vi "VI 1.vi"() -> ()   [LabVIEW 2020]
uses:
  <vilib>/express/express analysis/Spectral/Block/exnSpectralBlock spectral measurements RMS poly.vi
  <vilib>/express/express analysis/Spectral/Block/exnSpectralBlock spectral measurements RMS DDT.vi
  <vilib>/express/express analysis/Spectral/XNode/ExpressSpectralMeasurementsBlockNode.xnode
panel:
  out "Minimum":dbl
  out "Maksimum":dbl
  out "RMS":dbl
  out "Specific Harmonic Level":dbl
  out "THD":dbl
  out "SINAD":dbl
  out "Przebieg FFT":dynamicdata(graph)
  in  "Numer Harmonicznej":dbl=2.0 min=2.0 step=1.0
  in  "Faza 4":dbl min=0.0 step=0.1
  in  "Amplituda 4":dbl step=0.1
  in  "Numer Harmonicznej":dbl=2.0 min=2.0 step=1.0
  in  "Faza 3":dbl min=0.0 step=0.1
  in  "Amplituda 3":dbl step=0.1
  in  "Numer Harmonicznej":dbl=2.0 min=2.0 step=1.0
  in  "Faza 2":dbl min=0.0 step=0.1
  in  "Amplituda 2":dbl=0.1 step=0.1
  in  "Faza 1":dbl=0.1 min=0.0 step=0.1
  in  "Amplituda 1":dbl=0.1 step=0.1
  in  "Czestotliwosc Bazowa":dbl=1.0 min=1.0 step=0.1
  out "Przebieg Sygnalu":dynamicdata(graph)
  in  "Stop":bool
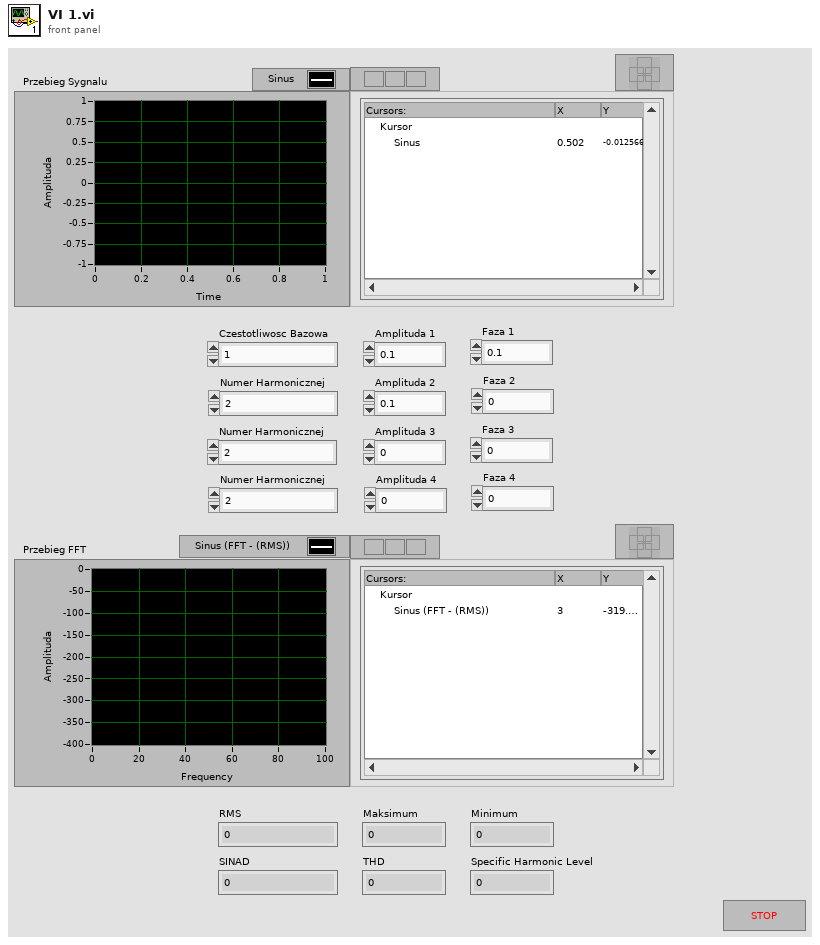
[diagram p1: front panel]
types:
  T1 = cluster{"averaging mode":u16, "weighting mode":u16, "number of averages":u32}
  T2 = cluster{"dB On (F)":bool, "unwrap phase (F)":bool, "convert to degree (F)":bool}
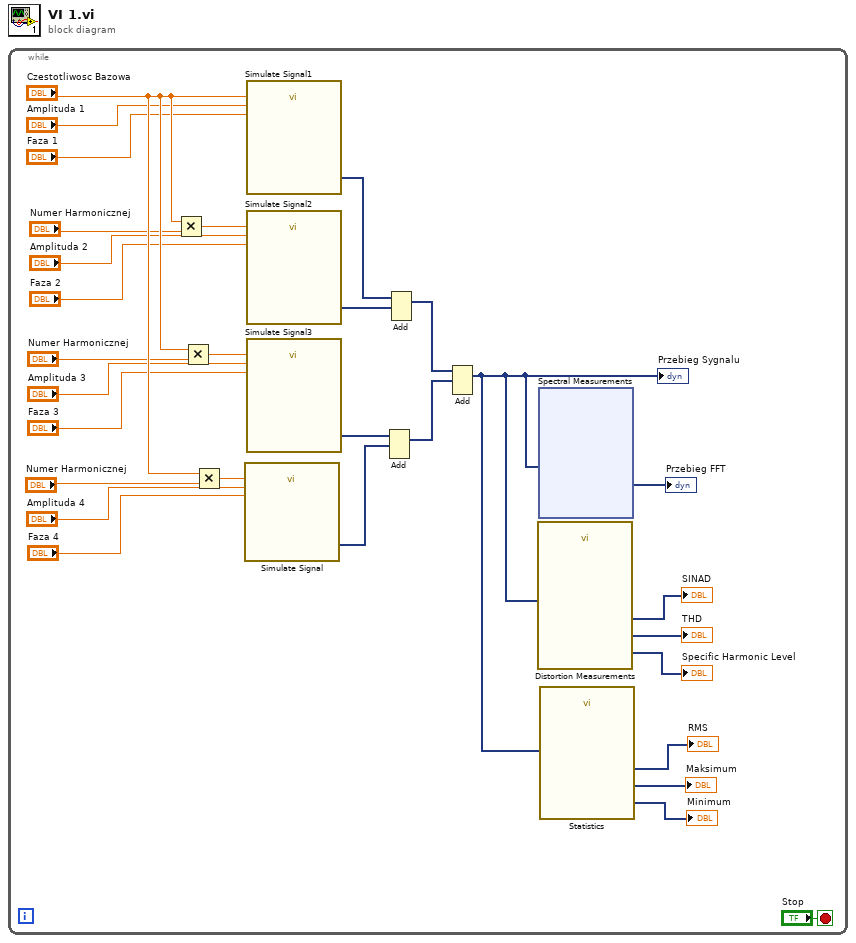
[diagram p0: block diagram]
diagram:
  n1 = while {
    stop <- "Stop" stop-if-true
    n2 = Multiply(x="Czestotliwosc Bazowa", y="Numer Harmonicznej") -> (x*y=w26:dbl)
    n3 = Multiply(x="Czestotliwosc Bazowa", y="Numer Harmonicznej") -> (x*y=w25:dbl)
    n4 = Multiply(x="Czestotliwosc Bazowa", y="Numer Harmonicznej") -> (x*y=w21:dbl)
    n5 = call "Simulate Signal"("Frequency"=w21, "Amplitude"="Amplituda 4", "Phase"="Faza 4") -> ("Harmoniczna3"=w23:dynamicdata)  [unwired: 11 in, 1 out]
    n6 = call "Simulate Signal1"("Frequency"="Czestotliwosc Bazowa", "Amplitude"="Amplituda 1", "Phase"="Faza 1") -> ("Sinus"=w29:dynamicdata)  [unwired: 11 in, 1 out]
    n7 = call "Simulate Signal2"("Frequency"=w26, "Amplitude"="Amplituda 2", "Phase"="Faza 2") -> ("Harmoniczna1"=w28:dynamicdata)  [unwired: 11 in, 1 out]
    n8 = call "Simulate Signal3"("Frequency"=w25, "Amplitude"="Amplituda 3", "Phase"="Faza 3") -> ("Harmoniczna2"=w24:dynamicdata)  [unwired: 11 in, 1 out]
    n9 = Add(1:w23, 2:w24) -> (0:w22:dynamicdata)  [unwired: 1 in, 1 out]
    n10 = Add(1:w28, 2:w29) -> (0:w27:dynamicdata)  [unwired: 1 in, 1 out]
    n11 = Add(1:w22, 2:w27) -> (0:w1:dynamicdata)  [unwired: 1 in, 1 out]
    "Przebieg Sygnalu" <- w1
    n12 = call "Distortion Measurements"("Signals"=w1) -> ("SINAD (dB)"=→"SINAD":dynamicdata, "Specific Harmonic"=→"Specific Harmonic Level":dynamicdata, "THD"=→"THD":dynamicdata)  [unwired: 7 in, 1 out]
    n13 = xnode "Spectral Measurements"("Signals"=w1) -> ("FFT - (RMS)"=→"Przebieg FFT":dynamicdata)  [unwired: 1 in, 2 out]
    n14 = call "Statistics"("Signals"=w1) -> ("RMS"=→"RMS":dynamicdata, "Minimum"=→"Minimum":dynamicdata, "Maximum"=→"Maksimum":dynamicdata)  [unwired: 23 in, 1 out]
  }
